vi "Close.vi"(11 "Custom Device in":refnum<class "Template.lvclass">) -> (0 "error out":errorcluster, 3 "Custom Device out":refnum<class "Template.lvclass">)   [LabVIEW 2026, in "Template.lvlib" / "Template.lvclass"]
uses:
  Template.lvclass
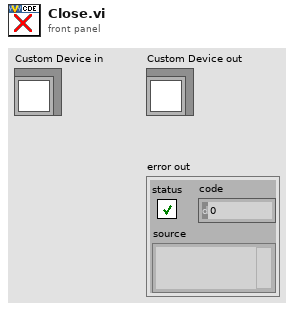
[diagram p1: front panel]
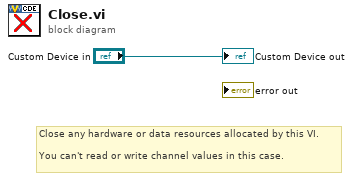
[diagram p0: block diagram]
diagram:
  # "Close any hardware or data resources allocated by this VI.\n\nYou can't read or write channel values in this case."
  "Custom Device out" <- "Custom Device in"
